vi "extractSingleCharacter.vi"(8 "error in (no error)":errorcluster, 10 "inputString":string, 11 "ILC in":refnum<class "ILC.lvclass">) -> (0 "error out":errorcluster, 1 "remainingString":string, 2 "extractedSegment":string, 3 "ILC out":refnum<class "ILC.lvclass">)   [LabVIEW 2015, in "ILCCommon.lvlib" / "ILC.lvclass"]
uses:
  <userlib>/Common/ILC/ILC/ILC.lvclass
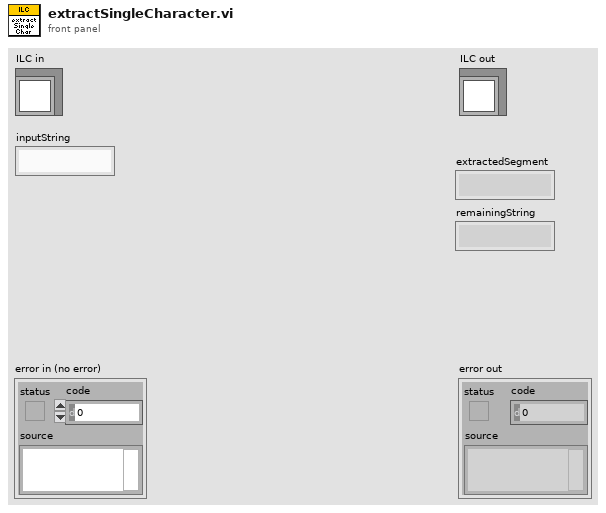
[diagram p1: front panel]
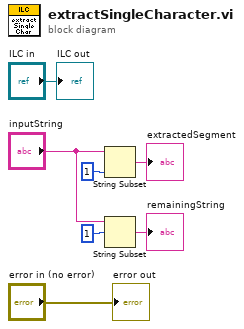
[diagram p0: block diagram]
diagram:
  n1 = String Subset(string="inputString", length (rest)=1 ("length (rest)")) -> (substring=→"extractedSegment":string)  [unwired: 1 in]
  n2 = String Subset(string="inputString", offset (0)=1) -> (substring=→"remainingString":string)  [unwired: 1 in]
  "error out" <- "error in (no error)"
  "ILC out" <- "ILC in"
